vi "Main.vi"(8 "error in (no error)":errorcluster, 11 "FactoryMethodDemo":refnum<class "ClientDemo.lvclass">) -> (0 "error out":errorcluster, 3 "FactoryMethodDemo":refnum<class "ClientDemo.lvclass">)   [LabVIEW 2020, in "FactoryMethod.lvlib" / "ParameterizedFactoryMethod.lvlib" / "ClientDemo.lvclass"]
uses:
  ClientDemo.lvclass
  MazeGame/API/TypeDef/MazeGameID.ctl
  MazeGame/MazeGame.lvclass
  GoFcommonClasses/Maze/Maze.lvclass
  Support/Class/ConsoleOutput.lvclass
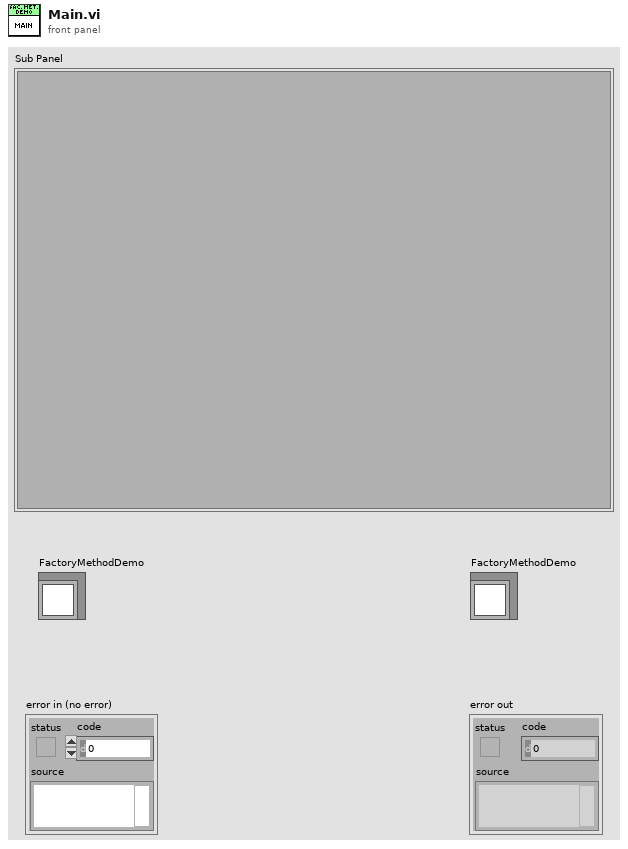
[diagram p1: front panel]
types:
  T1 = typedef "FactoryMethod.lvlib/ParameterizedFactoryMethod.lvlib/MazeGame.lvclass/MazeGameID.ctl" = enum16{"Normal", "Bombed", "Enchanted"}
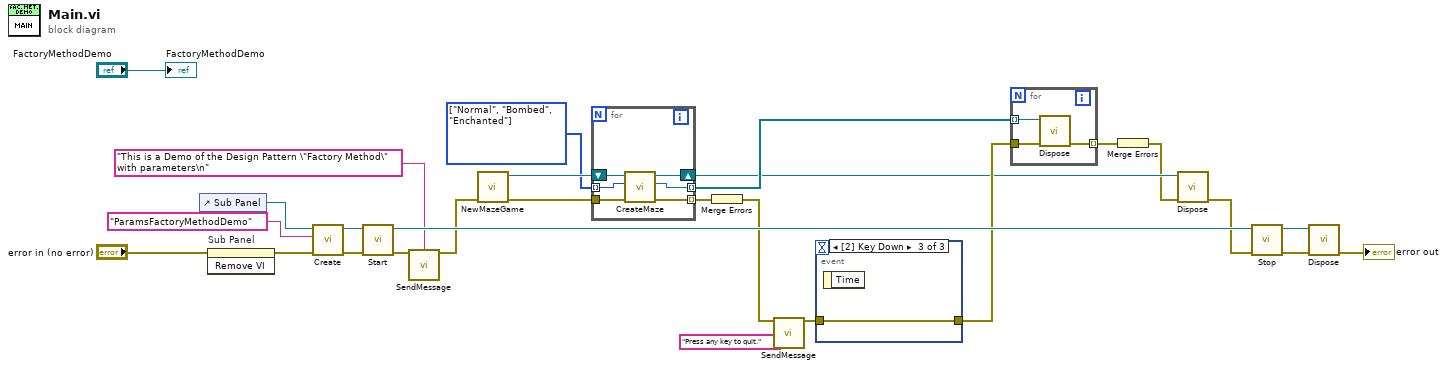
[diagram p0: block diagram]
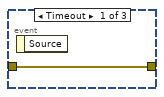
[diagram p2: hidden frame]
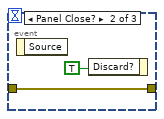
[diagram p3: hidden frame]
diagram:
  w4 = T1[] [enum."Normal", enum."Bombed", enum."Enchanted"] items=["Normal", "Bombed", "Enchanted"]
  n1 = control-ref of="Sub Panel"() -> (w19:refnum<vi>)
  n2 = invoke on="Sub Panel" class="SubPnl" method="Remove VI"(error in="error in (no error)") -> (error out=w20:errorcluster)  [unwired: 2 in, 2 out]
  n3 = call "Create.vi"("error in (no error)"=w20, "LoggerName"="ParamsFactoryMethodDemo", "SubPanelRef"=w19) -> ("error out"=w27:errorcluster, "ConsoleOutput out"=w26:refnum<class "ConsoleOutput.lvclass">)  [unwired: 7 in]
  n4 = call "Start.vi"("error in (no error)"=w27, "ConsoleOutput in"=w26) -> ("error out"=w21:errorcluster, "ConsoleOutput out"=w23:refnum<class "ConsoleOutput.lvclass">)  [unwired: 8 in]
  n5 = call "SendMessage.vi"("Message"="This is a Demo of the Design Pattern \"Factory Method\" with parameters\n" ("Data"), "error in (no error)"=w21) -> ("error out"=w13:errorcluster)  [unwired: 13 in]
  n6 = call "NewMazeGame.vi"("error in (no error)"=w13) -> ("error out"=w11:errorcluster, "MazeGame"=w12:refnum<class "MazeGame.lvclass">)  [unwired: 9 in]
  n7 = for {
    tunnel: [w30] -> w14 mode=indexing
    tunnel: w11 -> [w32]
    tunnel: [w29] -> w5 mode=indexing
    tunnel: w4 -> [w28] mode=indexing
    shift-right: [w31] -> w3
    shift-left: w12 -> [w33]
    n8 = call "CreateMaze.vi"("error in (no error)"=w32, "MazeGameID"=w28, "MazeGame"=w33) -> ("error out"=w30:errorcluster, "Maze"=w29:refnum<class "Maze.lvclass">, "MazeGame"=w31:refnum<class "MazeGame.lvclass">)  [unwired: 6 in]
  }
  n9 = Merge Errors(w14) -> (w7:errorcluster)
  n10 = call "SendMessage.vi"("Message"="Press any key to quit." ("Data"), "error in (no error)"=w7) -> ("error out"=w6:errorcluster)  [unwired: 13 in]
  n11 = event shown="[2] Key Down" {
    selector: _ -> [_ _ _]
    dyn-events: _ -> [_ _ _]
    timeout: _ -> [_ _ _]
    tunnel: w6 -> [w34 w36 w37]
    tunnel: [w34 w36 w37] -> w10
    event Timeout {
      n12 = event-data() -> ()  [unwired: 1 in, 1 out]
    }
    event Panel Close? {
      n13 = event-data() -> ()  [unwired: 1 in, 1 out]
      n14 = event-data("Discard?"=TRUE) -> ()  [unwired: 1 in, 1 out]
    }
    event Key Down {
      n15 = event-data() -> ()  [unwired: 1 in, 1 out]
    }
  }
  n16 = for {
    tunnel: w10 -> [w39]
    tunnel: [w38] -> w9 mode=indexing
    tunnel: w5 -> [w40] mode=indexing
    n17 = call-dynamic "Dispose.vi"("error in (no error)"=w39, "Maze"=w40) -> ("error out"=w38:errorcluster)  [unwired: 9 in]
  }
  n18 = Merge Errors(w9) -> (w2:errorcluster)
  n19 = call-dynamic "Dispose.vi"("error in (no error)"=w2, "ByRef"=w3) -> ("error out"=w1:errorcluster)  [unwired: 9 in]
  n20 = call "Stop.vi"("error in (no error)"=w1, "ConsoleOutput in"=w23) -> ("error out"=w16:errorcluster, "ConsoleOutput out"=w24:refnum<class "ConsoleOutput.lvclass">)  [unwired: 8 in]
  n21 = call "Dispose.vi"("error in (no error)"=w16, "ConsoleOutput in"=w24) -> ("error out"=→"error out":errorcluster)  [unwired: 9 in]
  "FactoryMethodDemo" <- "FactoryMethodDemo"
